vi "ctx get device id by index.vi"(10 "sensor_index":u32, 11 "context":u32) -> (2 "function return":i32, 3 "context out":u32)   [LabVIEW 2019, in "apdm.lvlib"]
doc: "APDM_EXPORT int32_t apdm_ctx_get_device_id_by_index(apdm_ctx_t context, const uint32_t sensor_index);"
uses:
  apdm.lvlib
  Lee Lab/CP FES Walking 2018/Code/Working/LabVIEW/apdm.dll
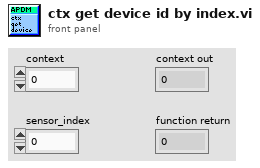
[diagram p1: front panel]
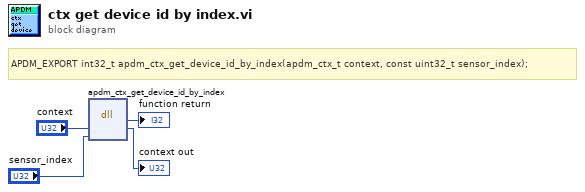
[diagram p0: block diagram]
diagram:
  # "APDM_EXPORT int32_t apdm_ctx_get_device_id_by_index(apdm_ctx_t context, const uint32_t sensor_index);"
  n1 = dll-call lib="C:/Users/jfalesi/Dropbox/Lee Lab/CP FES Walking 2018/Code/Working/LabVIEW/apdm.*" fn="apdm_ctx_get_device_id_by_index"("context"="context", "sensor_index"="sensor_index") -> (→"function return":i32, "context"=→"context out":u32)  [unwired: 4 in, 2 out]
